vi "Osciloscopio2.vi"() -> ()   [LabVIEW 2015]
uses:
  <vilib>/measure/NI_MABase.lvlib
panel:
  in  "Frecuencia\nTriangular":dbl(knob) scale=0.0..20.0
  in  "Amplitud\nTriangular":dbl(knob) scale=0.0..20.0
  in  "Frecuencia\nCuadrada":dbl(knob) scale=0.0..20.0
  in  "Amplitud\nCuadrada":dbl(knob) scale=0.0..20.0
  out "Waveform Graph":waveform(dbl)[](graph)
  in  "Frecuencia\nSenoidal":dbl(knob) scale=0.0..20.0
  in  "Amplitud\nSenoidal":dbl(knob) scale=0.0..20.0
  in  "stop":bool
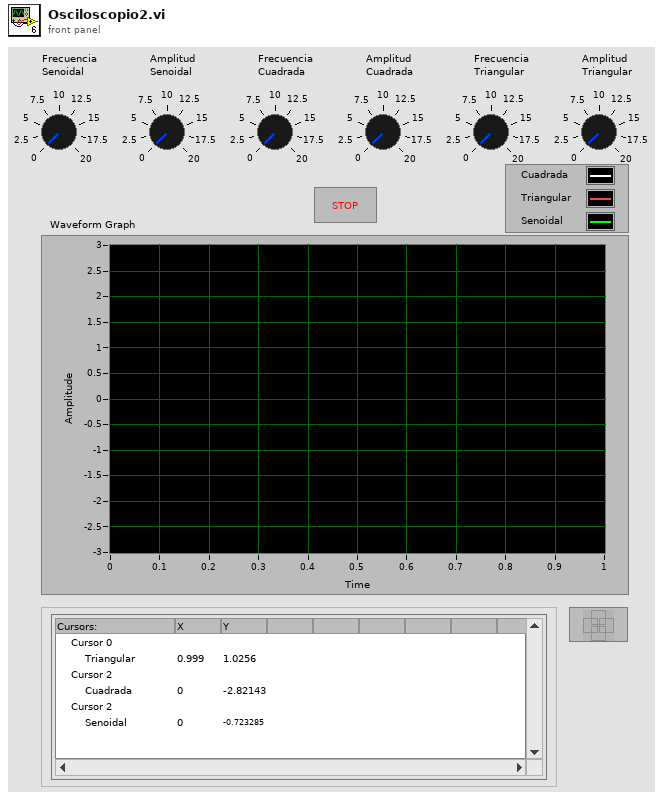
[diagram p1: front panel]
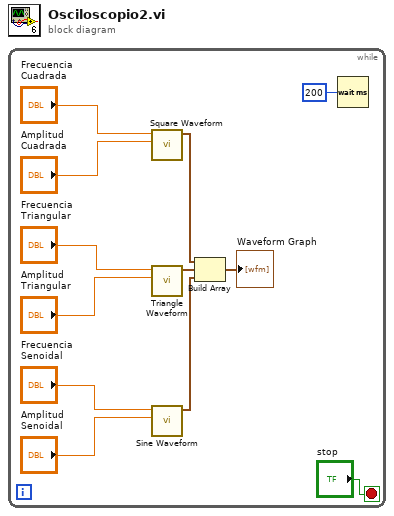
[diagram p0: block diagram]
diagram:
  n1 = while {
    stop <- "stop" stop-if-true
    n2 = call <vilib>:"Square Waveform.vi"("amplitude"="Amplitud\nCuadrada", "frequency"="Frecuencia\nCuadrada") -> ("signal out"=w4:waveform(dbl))  [unwired: 8 in, 1 out]
    n3 = call <vilib>:"Triangle Waveform.vi"("amplitude"="Amplitud\nTriangular", "frequency"="Frecuencia\nTriangular") -> ("signal out"=w3:waveform(dbl))  [unwired: 8 in, 1 out]
    n4 = call <vilib>:"Sine Waveform.vi"("amplitude"="Amplitud\nSenoidal", "frequency"="Frecuencia\nSenoidal") -> ("signal out"=w2:waveform(dbl))  [unwired: 8 in, 1 out]
    n5 = Build Array(w4, w3, w2) -> (→"Waveform Graph":waveform(dbl)[])
    n6 = Wait (ms)(milliseconds to wait=u32 200) -> ()  [unwired: 1 out]
  }
